vi "On File Open.vi"(8 "error in (no error)":errorcluster, 10 "Path":path, 11 "File Open Event Registrations in":T1[](array[typedef])) -> (0 "error out":errorcluster, 3 "File Open Event Registrations out":T1[](array[typedef]))   [LabVIEW 2015, in "Waveform Data Logger Engine.lvlib" / "Segmented Log.lvclass"]
uses:
  Segmented Log.lvclass
  File Open Event Registration.ctl
  File Open Event Data.ctl
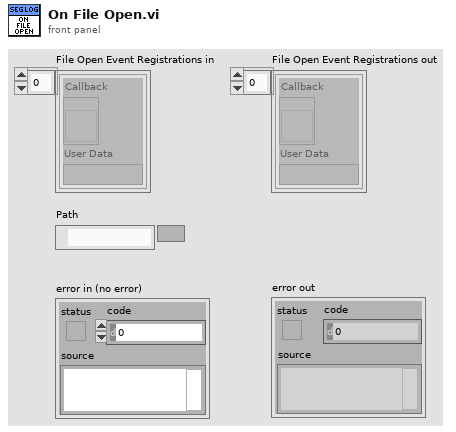
[diagram p1: front panel]
types:
  T1 = typedef "Waveform Data Logger Engine.lvlib/Segmented Log.lvclass/File Open Event Registration.ctl" = cluster{"Callback":refnum<vi>, "User Data":variant}
  T2 = typedef "Waveform Data Logger Engine.lvlib/Segmented Log.lvclass/File Open Event Data.ctl" = cluster{"File Path":path, "User Data":variant}
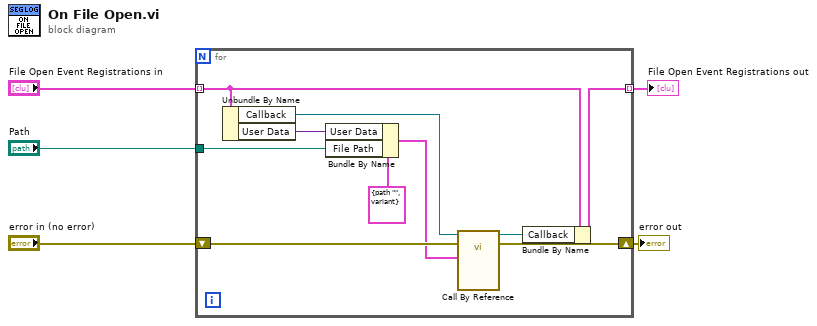
[diagram p0: block diagram]
diagram:
  n1 = for {
    tunnel: "File Open Event Registrations in" -> [w10] mode=indexing
    shift-right: [w11] -> w3
    shift-left: "error in (no error)" -> [w15]
    tunnel: [w9] -> w2 mode=indexing
    tunnel: "Path" -> [w6]
    n2 = Unbundle By Name(w10) -> ("Callback"=w14:refnum<vi>, "User Data"=w13:variant)
    n3 = Bundle By Name(cluster=T2 {"File Path"=path "", "User Data"=variant} ("File Open Event Data"), "User Data"=w13, "File Path"=w6) -> (w12:T2)
    n4 = call-by-ref "?"(reference=w14, error in=w15, "File Open Event Data"=w12) -> (reference out=w8:refnum<vi>, error out=w11:errorcluster)  [unwired: 11 in]
    n5 = Bundle By Name(cluster=w10, "Callback"=w8) -> (w9:T1)
  }
  "error out" <- w3
  "File Open Event Registrations out" <- w2
